vi "RESET.vi"(8 "error in (no error)":errorcluster, 11 "instrument handle":refnum<k15>) -> (0 "error out":errorcluster, 3 "instrument handle out":refnum<k15>)   [LabVIEW 2019]
uses:
  <instrlib>/niDigital/niDigital.llb/niDigital Burst Pattern (Burst Only).vi
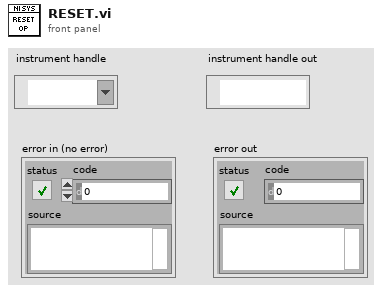
[diagram p1: front panel]
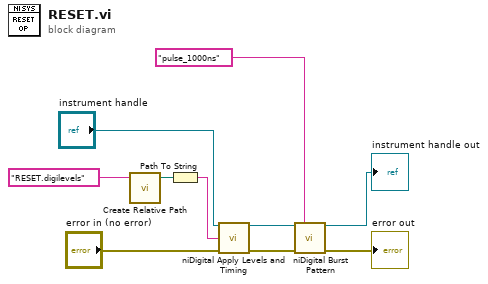
[diagram p0: block diagram]
diagram:
  n1 = call "Create Relative Path.vi"("file name"="RESET.digilevels") -> ("appended path"=w2:path)  [unwired: 4 in]
  n2 = Path To String(path=w2) -> (string=w5:string)
  n3 = call <instrlib>:"niDigital Apply Levels and Timing.vi"("instrument handle"="instrument handle", "levels sheet"=w5, "error in"="error in (no error)") -> ("instrument handle out"=w3:refnum<k15>, "error out"=w4:errorcluster)  [unwired: 11 in]
  n4 = call-poly <instrlib>:"niDigital Burst Pattern.vi"("instrument handle"=w3, "start label"="pulse_1000ns", "error in"=w4) -> ("instrument handle out"=→"instrument handle out":refnum<k15>, "error out"=→"error out":errorcluster)  [unwired: 11 in]
